vi "Rohdaten abholen.vi"(8 "error in (no error)":errorcluster caption="Fehler (Eingang, kein Fehler)", 11 "Temp. Messzelle G-nr.":i32) -> (0 "error out":errorcluster caption="Fehler (Ausgang)")   [LabVIEW 2015, in "Linearisierung V2.lvlib"]
uses:
  Linearisierung V2.lvlib
  Messdaten/Messdaten.lvlib
  Messdaten/Aktionen FGV Messdaten.ctl
  Messdaten/Gewichtung (Stichprobe).ctl
  Seiten/FT-IR/FT-IR.lvlib
  Seiten/FT-IR/Aktionen EVID-Codes.ctl
  Seiten/FT-IR/FGV FT-IR Aktionen.ctl
  Aktion Lin Daten aufarbeiten.ctl
  Aktion FGV Rohmesswerte sammeln.ctl
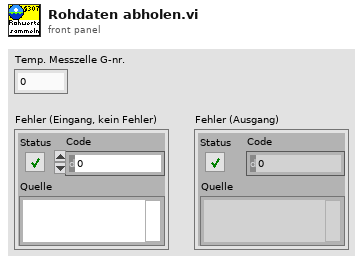
[diagram p1: front panel]
types:
  T1 = typedef "Linearisierung V2.lvlib/Aktion Lin Daten aufarbeiten.ctl" = enum16{"lesen", "Protkolldaten", "speichern", "laden", "EPA auswerten", "Tabelle schreiben", "Lin auswerten", "Tab init", "Stufentabelle", "EPA aktiviert", "Nachbehandlung laden", "Tabelle löschen", "Istwerte löschen", "Zeile löschen", "Zeile einfügen", "LIN aktiviert", "LIN/EPA aktiv laden"}
  T2 = typedef "Neue Linearisierung.lvlib/Lin-Polynom Daten.ctl" = cluster{"Messgerät":string, "Kalibrator (Gasteiler)":string, "Bearbeiter/in":string, "Komponente":string, "Zeitstempel":timestamp, "F_max gefordert (%)":sgl, "F_max in %":sgl, "F_max in ppm":sgl, "Vorschlag Ordnung":i32, "Polynom OK":bool, "Polynomkoeff.":sgl[], "Prüfgas Konzentration":sgl, "Pfad1":string, "Pfad_LIN":string, "Gasnummer:":u8, "Komponentenauswahl":T3, "Verdünnungsgas":T5, "Zeitdauer Stufe":T6, "Anzahl Stufen":T6, "F_max in % EPA":sgl, "F_max in ppm EPA":sgl, "F_max in % LIN":sgl, "F_max in ppm LIN":sgl, "Punkte umkehren":bool, "EPA Optionsfeld":T7}
  T3 = typedef "Neue Linearisierung.lvlib/KomponentenArray.ctl" = cluster{"Komponente:":T4, "Konzentration":sgl}[]
  T4 = typedef "Auswahlfeld.ctl" = u16
  T5 = typedef "Neue Linearisierung.lvlib/Gasteiler.lvlib/Prüfgas in.ctl" = u16
  T6 = typedef "Zahlen-Eingabefeld.ctl" = sgl
  T7 = typedef "Neue Linearisierung.lvlib/EPA Optionsfeld.ctl" = enum32{"Istwert", "Rohwert", "Linearisierter Wert"}
  T8 = cluster{"Aktuelle Messwert":dbl, "Aktuelle Rohwert":dbl, "Deviation":dbl, "Temp":dbl, "Druck":dbl}
  T9 = typedef "Messdaten.lvlib/Gewichtung (Stichprobe).ctl" = enum16{"Sample", "Population"}
  T10 = typedef "Linearisierung V2.lvlib/Aktion FGV Rohmesswerte sammeln.ctl" = enum16{"lesen", "schreiben", "löschen", "Sollwert HovaCal"}
  T11 = typedef "FT-IR.lvlib/FGV FT-IR Aktionen.ctl" = enum16{"lesen", "NOG setzen", "NOS setzen", "Initialisieren", "speichern", "ALLES setzen", "FT-IR Spektrum loggen", "Komm Stoppen"}
  T12 = typedef "FT-IR.lvlib/Aktionen EVID-Codes.ctl" = enum16{"lesen", "setzen", "laden", "speichern", "1Hz/5Hz", "Smoothing"}
  T13 = typedef "Messdaten.lvlib/Aktionen FGV Messdaten.ctl" = enum16{"lesen", "schreiben", "löschen", "Mittelwerte", "Komponente"}
  T14 = typedef "FT-IR.lvlib/1Hz-5Hz Geraet.ctl" = u16
  T15 = typedef "Neue Linearisierung.lvlib/Eingabetabelle.ctl" = string[][]
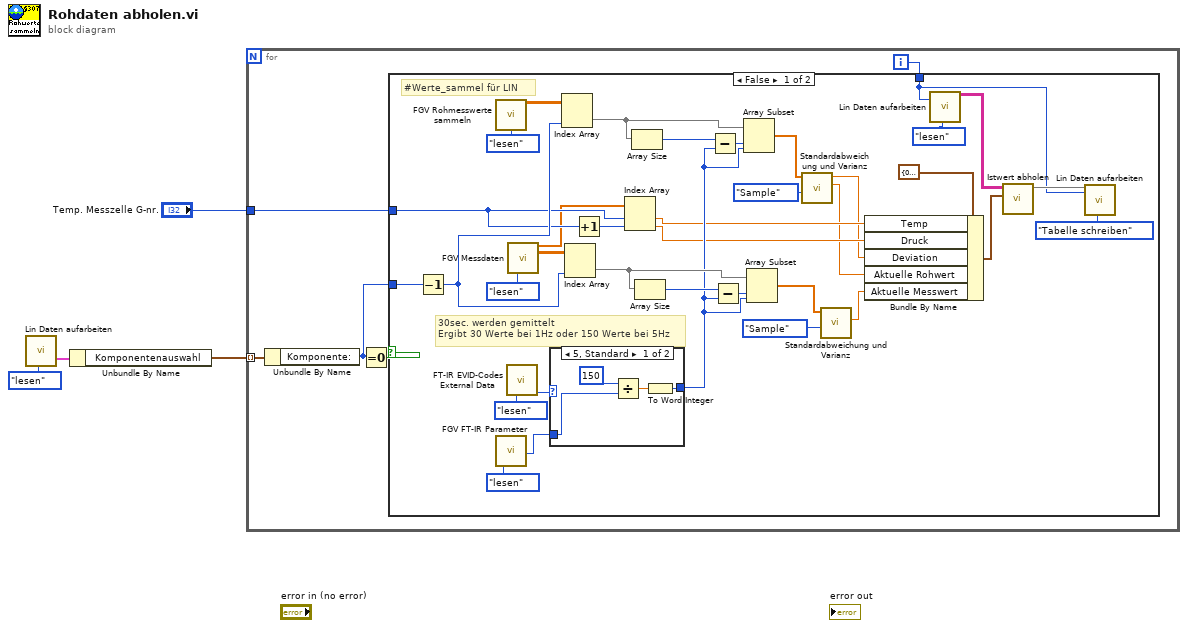
[diagram p0: block diagram]
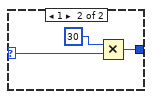
[diagram p2: hidden frame]
diagram:
  n1 = call "Lin Daten aufarbeiten.vi"("Aktionen"=Aktion_Lin_Daten_aufarbeiten."lesen") -> ("Lin-Polynom"=w3:T2)  [unwired: 11 in, 7 out]
  n2 = Unbundle By Name(w3) -> ("Komponentenauswahl"=w2:T3)
  n3 = for {
    tunnel: w2 -> [w9] mode=indexing
    tunnel: "Temp. Messzelle G-nr." -> [w5]
    i -> [w6]
    n4 = Unbundle By Name(w9) -> ("Komponente:"=w7:T4)
    n5 = Equal To 0?(x=w7) -> (x = 0?=w8:bool)
    n6 = case shown="False" w8 {
      tunnel: w7 -> [w29 _]
      tunnel: w6 -> [w20 _]
      tunnel: w5 -> [w18 _]
      frame False {
        # "#Werte_sammel für LIN"
        # "30sec. werden gemittelt\nErgibt 30 Werte bei 1Hz oder 150 Werte bei 5Hz"
        n7 = Decrement(x=w29) -> (x-1=w25:T4)
        n8 = call "FGV Rohmesswerte sammeln.vi"("Aktion"=Aktion_FGV_Rohmesswerte_sammeln."lesen") -> ("Rohmessdaten"=w30:sgl[][])  [unwired: 11 in, 3 out]
        n9 = call "FGV FT-IR Parameter.vi"("Aktion"=FGV_FT-IR_Aktionen."lesen") -> ("NoOfScan"=w45:u32)  [unwired: 11 in, 7 out]
        n10 = call "FT-IR EVID-Codes External Data.vi"("Aktionen"=Aktionen_EVID-Codes."lesen") -> ("1Hz/5Hz Gerät"=w44:T14)  [unwired: 9 in, 5 out]
        n11 = call "FGV Messdaten.vi"("Aktionen"=Aktionen_FGV_Messdaten."lesen") -> ("Aktuelle Messwerte"=w17:sgl[], "Messdaten"=w39:sgl[][])  [unwired: 6 in, 7 out]
        n12 = case shown="5, Standard" w44 {
          selector: w44 -> [_ w50]
          tunnel: [w46 w51] -> w26
          tunnel: w45 -> [w48 _]
          frame 5, Default {
            n13 = Divide(x=150, y=w48) -> (x/y=w47:dbl)
            n14 = To Word Integer(number=w47) -> (16bit integer=w46:i16)
          }
          frame 1 {
            n15 = Multiply(x=30, y=w50) -> (x*y=w51:i32)
          }
        }
        n16 = Index Array(array=w30, index (col)=w25) -> (element=w33:sgl[])  [unwired: 1 in]
        n17 = Index Array(array=w39, index (col)=w25) -> (element=w40:sgl[])  [unwired: 1 in]
        n18 = Increment(x=w18) -> (x+1=w19:i32)
        n19 = Index Array(array=w17, index #1=w18, index #2=w19) -> (element #1=w14:sgl, element #2=w13:sgl)
        n20 = Array Size(array=w33) -> (size(s)=w32:i32)
        n21 = Array Size(array=w40) -> (size(s)=w41:i32)
        n22 = Subtract(x=w32, y=w26) -> (x-y=w34:i32)
        n23 = Subtract(x=w41, y=w26) -> (x-y=w36:i32)
        n24 = Array Subset(array=w33, index=w34, length=w26) -> (w27:sgl[])
        n25 = Array Subset(array=w40, index=w36, length=w26) -> (w42:sgl[])
        n26 = call "Standardabweichung und Varianz.vi"("Gewichtung (Stichprobe)"=Gewichtung_(Stichprobe)."Sample", "X"=w27) -> ("Mittelwert"=w11:sgl, "Standardabweichung"=w12:sgl)  [unwired: 7 in, 1 out]
        n27 = call "Standardabweichung und Varianz.vi"("Gewichtung (Stichprobe)"=Gewichtung_(Stichprobe)."Sample", "X"=w42) -> ("Mittelwert"=w10:sgl)  [unwired: 7 in, 2 out]
        n28 = Bundle By Name(cluster=T8 {"Aktuelle Messwert"=0.0, "Aktuelle Rohwert"=0.0, "Deviation"=0.0, "Temp"=0.0, "Druck"=0.0} ("Eingangswerte"), "Temp"=w14, "Druck"=w13, "Deviation"=w12, "Aktuelle Rohwert"=w11, "Aktuelle Messwert"=w10) -> (w15:T8)
        n29 = call "Lin Daten aufarbeiten.vi"("Index (Seite)"=w20, "Aktionen"=Aktion_Lin_Daten_aufarbeiten."lesen") -> ("Eingabetabelle"=w23:T15)  [unwired: 10 in, 7 out]
        n30 = call "Istwert abholen.vi"("Eingangswerte"=w15, "Gasindex"=w23) -> (3:w21)  [unwired: 9 in]
        n31 = call "Lin Daten aufarbeiten.vi"("Eingabetabelle"=w21, "Index (Seite)"=w20, "Aktionen"=Aktion_Lin_Daten_aufarbeiten."Tabelle schreiben") -> ()  [unwired: 9 in, 8 out]
      }
      frame True {
        # "Wenn kein Gas eingestellt ist, dann auch nichts\nmachen"
      }
    }
  }
